vi "CenterToRectangle.vi"(9 "hight":i32, 10 "width":i32, 11 "center":cluster{i32, i32}) -> (3 "rectangle":cluster{i32, i32, i32, i32}={253, 74, 453, 274})   [LabVIEW 2011]
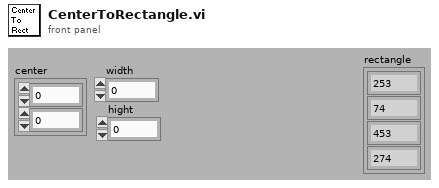
[diagram p1: front panel]
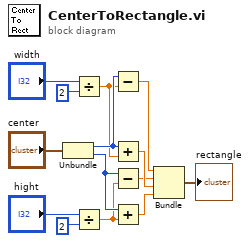
[diagram p0: block diagram]
diagram:
  n1 = Unbundle("center") -> (w10:i32, w4:i32)
  n2 = Divide(x="width", y=2) -> (x/y=w9:dbl)
  n3 = Divide(x="hight", y=2) -> (x/y=w3:dbl)
  n4 = Subtract(x=w10, y=w9) -> (x-y=w11:dbl)
  n5 = Add(x=w10, y=w9) -> (x+y=w8:dbl)
  n6 = Subtract(x=w4, y=w3) -> (x-y=w5:dbl)
  n7 = Add(x=w4, y=w3) -> (x+y=w2:dbl)
  n8 = Bundle(w11, w5, w8, w2) -> (→"rectangle":cluster{dbl, dbl, dbl, dbl})  [unwired: 1 out]
